vi "Destroy Events.vi"(8 "error in (no error)":errorcluster, 11 "DAQ":refnum<class "DAQ.lvclass">) -> (0 "error out":errorcluster, 3 "DAQ":refnum<class "DAQ.lvclass">)   [LabVIEW 2022 SP3, in "DAQ.lvclass"]
doc: "Developed by Kevin Thompson\nkevin@thompsonengineering.net\n\nCopyright 2018-2020\nThompson Engineering, LLC"
uses:
  DAQ.lvclass
  DAQ.lvclass/DAQ.ctl
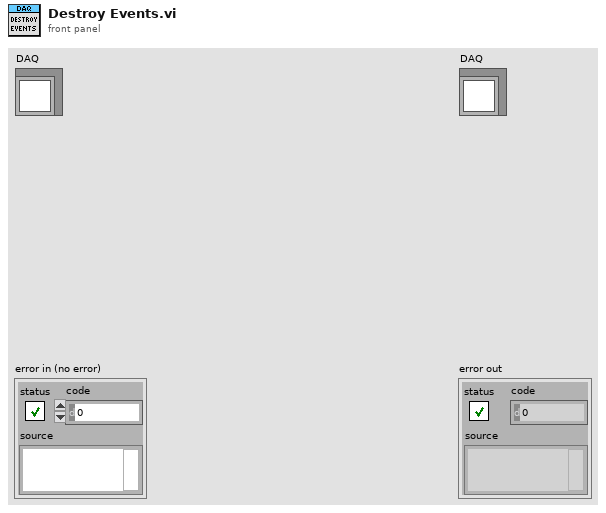
[diagram p1: front panel]
types:
  T1 = typedef "DAQ.lvclass/TD PublicEvents--cluster.ctl" = cluster{"DaqOutputCmd Ev":refnum<user-event>, "stop process":refnum<user-event>, "DAQ.AsyncCmd Event":refnum<user-event>, "DAQStateChanged Event":refnum<user-event>, "DAQ.AsyncMsg Event":refnum<user-event>, "DAQ_DO_StatusEvent":refnum<user-event>, "DIStateChangeEv":refnum<user-event>}
  T2 = cluster{"DAQ.AsyncMsg Event":refnum<user-event>, "DaqOutputCmd Ev":refnum<user-event>, "DAQ.AsyncCmd Event":refnum<user-event>, "DAQStateChanged Event":refnum<user-event>, "DAQ_DO_StatusEvent":refnum<user-event>, "DIStateChangeEv":refnum<user-event>}
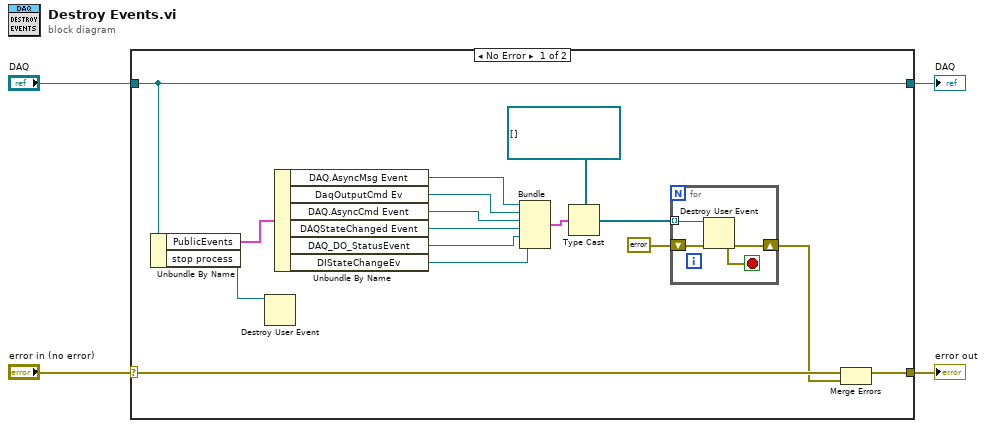
[diagram p0: block diagram]
diagram:
  n1 = case shown="No Error" "error in (no error)" {
    selector: "error in (no error)" -> [w14 w25]
    tunnel: [w15 w25] -> w3
    tunnel: [w20 w24] -> w1
    tunnel: "DAQ" -> [w20 w24]
    frame No Error {
      n2 = Unbundle By Name(w20) -> ("PublicEvents"=w8:T1, "stop process"=w19:refnum<user-event>)
      n3 = Destroy User Event(user event=w19) -> ()  [unwired: 1 in, 1 out]
      n4 = Unbundle By Name(w8) -> ("DAQ.AsyncMsg Event"=w7:refnum<user-event>, "DaqOutputCmd Ev"=w11:refnum<user-event>, "DAQ.AsyncCmd Event"=w10:refnum<user-event>, "DAQStateChanged Event"=w9:refnum<user-event>, "DAQ_DO_StatusEvent"=w6:refnum<user-event>, "DIStateChangeEv"=w5:refnum<user-event>)
      n5 = Bundle("DAQ.AsyncMsg Event"=w7, "DaqOutputCmd Ev"=w11, "DAQ.AsyncCmd Event"=w10, "DAQStateChanged Event"=w9, "DAQ_DO_StatusEvent"=w6, "DIStateChangeEv"=w5) -> (w17:T2)  [unwired: 1 in]
      n6 = Type Cast(type=refnum<user-event>[] [], x=w17) -> (*(type *) &x=w16:refnum<user-event>[])
      n7 = for {
        tunnel: w16 -> [w23] mode=indexing
        shift-right: [w21] -> w13
        shift-left: errorcluster {"status"=FALSE, "code"=0, "source"=""} ("error out") -> [w22]
        stop <- w21 stop-if-true
        n8 = Destroy User Event(user event=w23, error in=w22) -> (error out=w21:errorcluster)
      }
      n9 = Merge Errors(w14, w13) -> (w15:errorcluster)
    }
    frame Error {
    }
  }
  "error out" <- w3
  "DAQ" <- w1
